vi "Write Data.vi"(8 "error in (no error)":errorcluster, 10 "DatasFiles.DataWrite":variant, 11 "Masterv2 in":refnum<class "Masterv2.lvclass">) -> (0 "error out":errorcluster, 3 "Masterv2 out":refnum<class "Masterv2.lvclass">)   [LabVIEW 2014, in "Main Libraryv2.lvlib" / "Masterv2.lvclass"]
uses:
  Master/Masterv2.lvclass
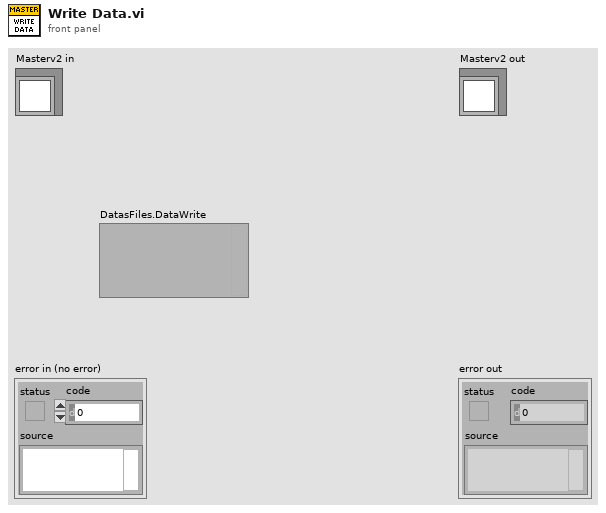
[diagram p1: front panel]
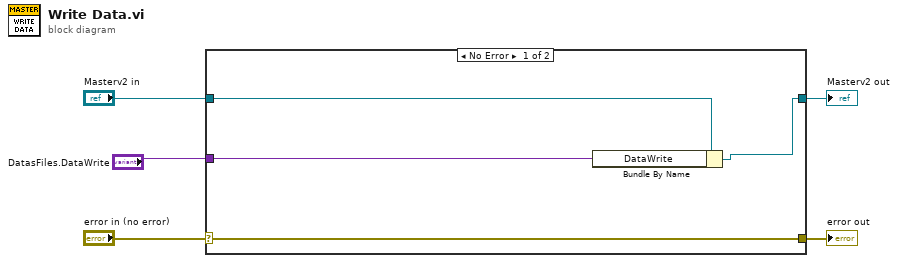
[diagram p0: block diagram]
diagram:
  n1 = case shown="No Error" "error in (no error)" {
    selector: "error in (no error)" -> [w9 w11]
    tunnel: [w9 w11] -> w4
    tunnel: [w7 w10] -> w2
    tunnel: "Masterv2 in" -> [w8 w10]
    tunnel: "DatasFiles.DataWrite" -> [w6 _]
    frame No Error {
      n2 = Bundle By Name(cluster=w8, "DataWrite"=w6) -> (w7:refnum<class "Masterv2.lvclass">)
    }
    frame Error {
    }
  }
  "error out" <- w4
  "Masterv2 out" <- w2
